vi "fin.vi"() -> ()   [LabVIEW 2018]
panel:
  out "Position (mm)":cluster{"X":dbl, "Y":dbl, "Theta":dbl}
  in  "error in":errorcluster
  in  "Position":cluster{"X":dbl, "Y":dbl, "Theta":dbl}
  out "range Out":dbl[](array[numeric])
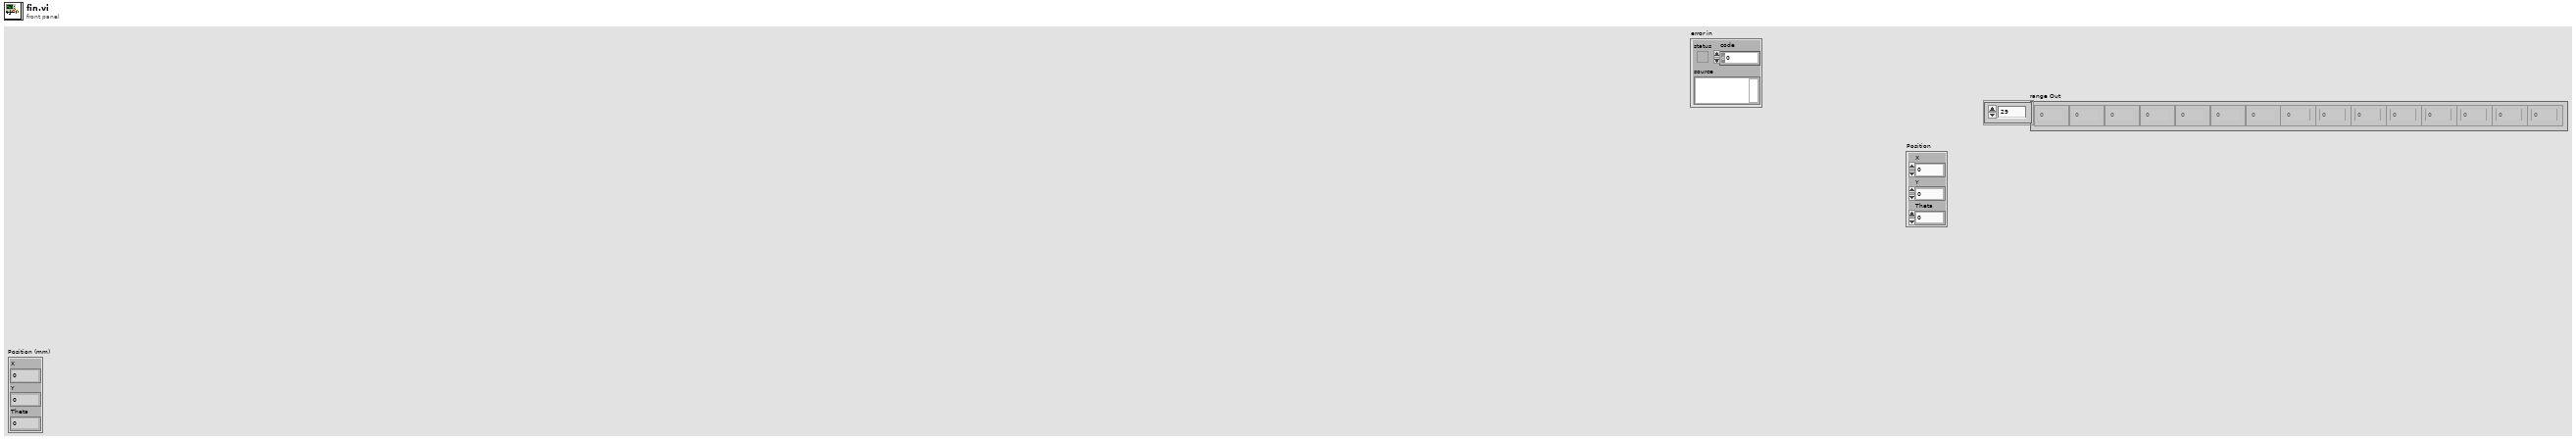
[diagram p1: front panel]
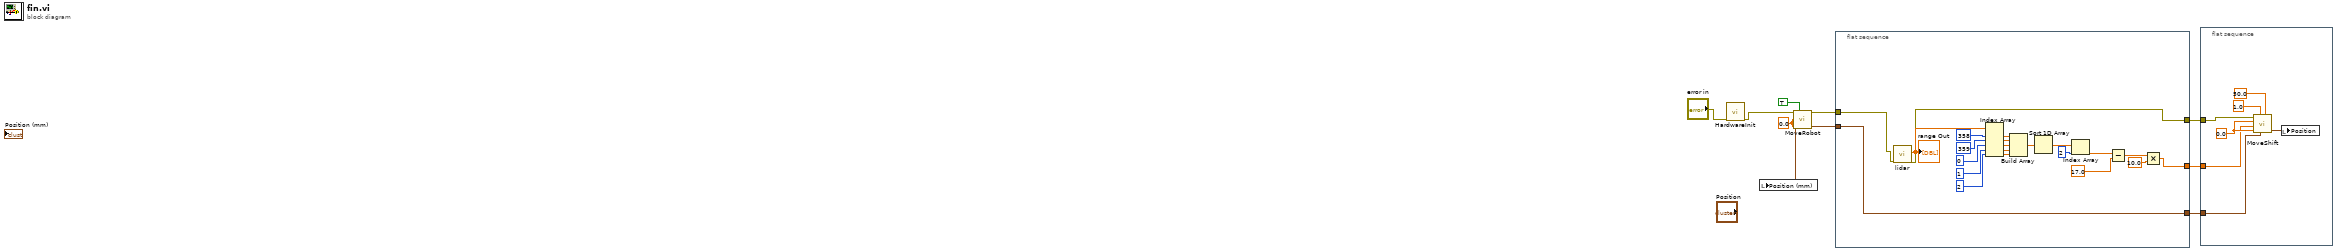
[diagram p0: block diagram]
diagram:
  w8 = 0.0 ("y (mm/s)")
  n1 = call "HardwareInit.vi"("Error/Flow In"="error in") -> ("error out"=w1:errorcluster)  [unwired: 10 in]
  n2 = call "MoveRobot.vi"("Error/Flow In"=w1, "Reset"=TRUE, "x (mm/s)"=w8, "y (mm/s)"=w8, "theta (rad/s)"=w8) -> ("Error/Flow Out"=w7:errorcluster, "Position"=w4:cluster{"X":dbl, "Y":dbl, "Theta":dbl})  [unwired: 9 in]
  n3 = local write "Position (mm)"(w4) -> ()
  n4 = flat-sequence {
    tunnel: w7 -> [w13]
    tunnel: [w12] -> w6
    tunnel: [w11] -> w5
    tunnel: w4 -> [w11]
    tunnel: [w10] -> w3
    frame #0 {
      n5 = call "lidar.vi"("error in (no error)"=w13) -> ("error out"=w12:errorcluster, "range Out"=w30:dbl[])  [unwired: 8 in, 1 out]
      "range Out" <- w30
      n6 = Index Array(array=w30, index #1=358 ("index"), index #2=359 ("index"), index #3=0 ("index"), index #4=1 ("index"), index #5=2 ("index")) -> (element #1=w24:dbl, element #2=w23:dbl, element #3=w22:dbl, element #4=w21:dbl, element #5=w20:dbl)
      n7 = Build Array(w24, w23, w22, w21, w20) -> (w19:dbl[])
      n8 = Sort 1D Array(array=w19) -> (sorted array=w18:dbl[])
      n9 = Index Array(array=w18, index=2) -> (element=w16:dbl)
      n10 = Subtract(x=w16, y=17.0) -> (x-y=w15:dbl)
      n11 = Multiply(x=w15, y=10.0) -> (x*y=w10:dbl)
    }
  }
  n12 = flat-sequence {
    tunnel: w6 -> [w34]
    tunnel: w5 -> [w33]
    tunnel: w3 -> [w32]
    frame #0 {
      w36 = 0.0 ("x shift")
      n13 = call "MoveShift.vi"("max speed"=50.0, "Position"=w33, "Precision"=1.0, "theta"=w36, "y shift"=w32, "x shift"=w36, "Error/Flow In"=w34) -> ("Position Out"=w35:cluster{"X":dbl, "Y":dbl, "Theta":dbl})  [unwired: 3 in, 1 out]
      n14 = local write "Position"(w35) -> ()
    }
  }
